vi "Prompt for Step--Init UI.vi"(8 "error in (no error)":errorcluster, 10 "Control Ref Map":map{string, refnum<vi>}(c390), 11 "Timing Action in":refnum<class "Timing Action.lvclass">) -> (0 "error out":errorcluster, 3 "Timing Action out":refnum<class "Timing Action.lvclass">)   [LabVIEW 2020, in "MacroAssert.lvlib" / "Timing Action.lvclass"]
doc: "Initializes the user interface within the \"Prompt for Step\" VI."
uses:
  Timing Action.lvclass
  af30d547-0726-4784-b602-959716fec50c.vi
  bffebe10-a113-4901-af85-4519943715b4.vi
  Support/Get Control Reference by Label (1D STR).vi
  <vilib>/Utility/error.llb/Error Cluster From Error Code.vi
  Action Step/Action Step.lvclass
  MacroAssert.lvlib
  SubVIs/Custom Errors/Custom Errors.lvlib
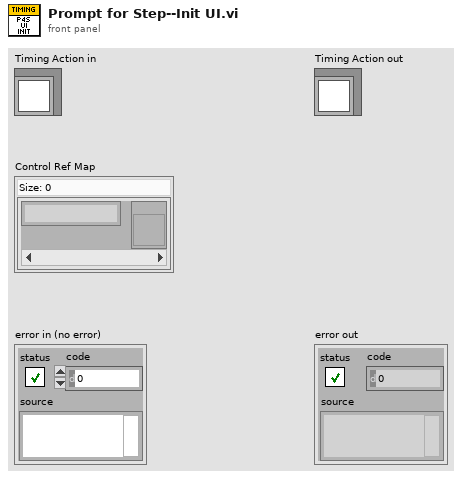
[diagram p1: front panel]
types:
  T1 = typedef "MacroAssert.lvlib/Timing Action.lvclass/Timing Action Type.ctl" = enum16{"Wait", "Wait Until"}
  T2 = typedef "MacroAssert.lvlib/Timing Action.lvclass/Time Unit.ctl" = enum16{"milliseconds", "seconds", "minutes"}
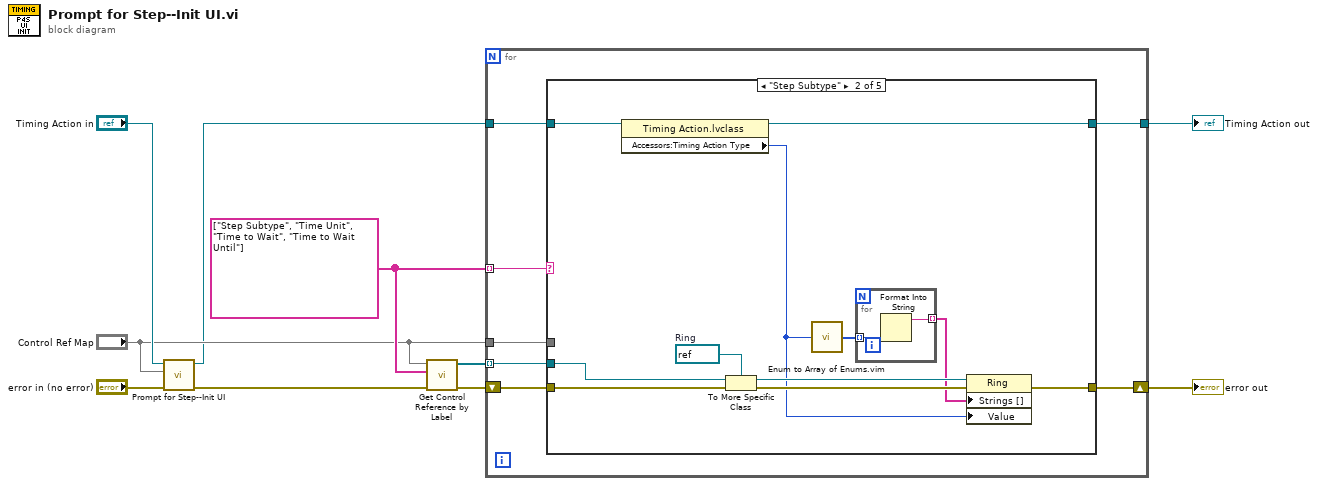
[diagram p0: block diagram]
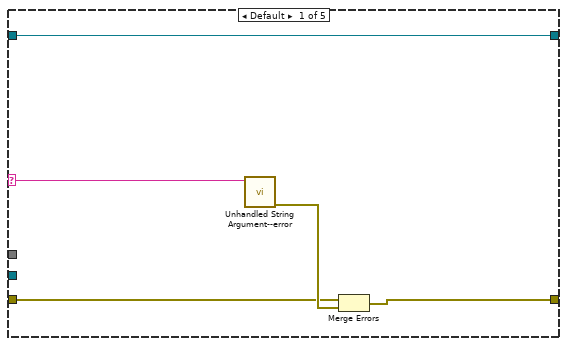
[diagram p2: hidden frame]
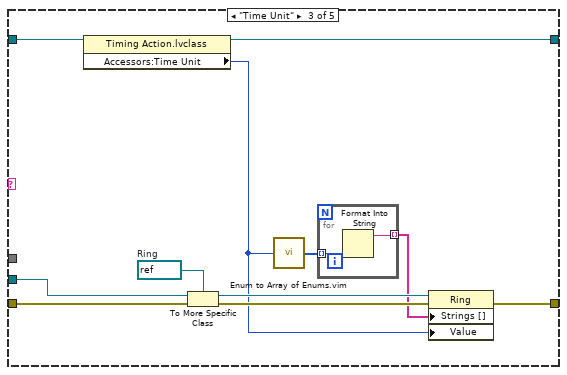
[diagram p3: hidden frame]
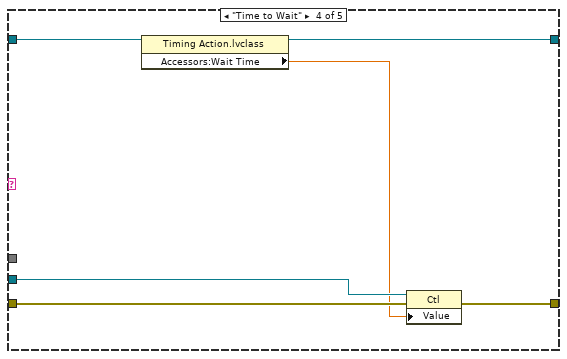
[diagram p4: hidden frame]
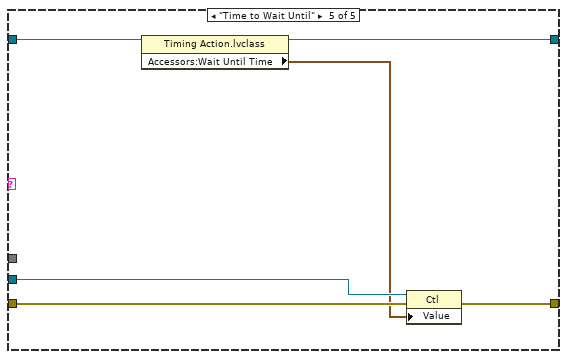
[diagram p5: hidden frame]
diagram:
  w9 = string[] ["Step Subtype", "Time Unit", "Time to Wait", "Time to Wait Until"]
  n1 = call-parent "Prompt for Step--Init UI.vi"("error in (no error)"="error in (no error)", "Control Ref Map"="Control Ref Map", "Step in"="Timing Action in") -> ("error out"=w4:errorcluster, "Step out"=w1:refnum<class "Timing Action.lvclass">)  [unwired: 7 in]
  n2 = call-poly "Get Control Reference by Label.vi"("error in (no error)"=w4, "Control Names"=w9, "Control Ref Map"="Control Ref Map") -> ("error out"=w10:errorcluster, "Control Refs"=w8:refnum<vi>[])  [unwired: 6 in, 1 out]
  n3 = for {
    tunnel: w1 -> [w15]
    tunnel: [w13] -> w5
    tunnel: w9 -> [w16] mode=indexing
    tunnel: w8 -> [w14] mode=indexing
    shift-right: [w12] -> w7
    shift-left: w10 -> [w17]
    tunnel: "Control Ref Map" -> [w11]
    n4 = case shown="\"Step Subtype\"" w16 {
      selector: w16 -> [w18 _ _ _ _]
      tunnel: w17 -> [w20 w26 w39 w51 w57]
      tunnel: w15 -> [w22 w27 w40 w54 w60]
      tunnel: w14 -> [_ w25 w38 w52 w58]
      tunnel: [w22 w23 w36 w53 w59] -> w13
      tunnel: [w19 w24 w37 w49 w55] -> w12
      tunnel: w11 -> [_ _ _ _ _]
      frame Default {
        n5 = call "Unhandled String Argument--error.vi"("Argument"=w18) -> ("error out"=w21:errorcluster)  [unwired: 10 in]
        n6 = Merge Errors(w20, w21) -> (w19:errorcluster)
      }
      frame "Step Subtype" {
        w30 = refnum<vi> refnum  # Ring
        n7 = property class="Timing Action.lvclass"(reference=w27) -> (reference out=w23:refnum<class "Timing Action.lvclass">, "Accessors:Timing Action Type"=w29:T1)  [unwired: 1 in, 1 out]
        n8 = To More Specific Class(target class=w30, reference=w25, error in=w26) -> (specific class reference=w33:refnum<vi>, error out=w31:errorcluster)
        n9 = call "Enum to Array of Enums.vim"("enum"=w29) -> ("array of enums"=w32:T1[])
        n10 = for {
          tunnel: w32 -> [w35] mode=indexing
          tunnel: [w34] -> w28 mode=indexing
          n11 = Format Into String(w35) -> (resulting string=w34:string)  [unwired: 3 in, 1 out]
        }
        n12 = property class="Ring"(reference=w33, error in=w31, "Strings []"=w28, "Value"=w29) -> (error out=w24:errorcluster)  [unwired: 1 out]
      }
      frame "Time Unit" {
        w43 = refnum<vi> refnum  # Ring
        n13 = property class="Timing Action.lvclass"(reference=w40) -> (reference out=w36:refnum<class "Timing Action.lvclass">, "Accessors:Time Unit"=w42:T2)  [unwired: 1 in, 1 out]
        n14 = To More Specific Class(target class=w43, reference=w38, error in=w39) -> (specific class reference=w46:refnum<vi>, error out=w44:errorcluster)
        n15 = call "Enum to Array of Enums.vim"("enum"=w42) -> ("array of enums"=w45:T2[])
        n16 = for {
          tunnel: w45 -> [w48] mode=indexing
          tunnel: [w47] -> w41 mode=indexing
          n17 = Format Into String(w48) -> (resulting string=w47:string)  [unwired: 3 in, 1 out]
        }
        n18 = property class="Ring"(reference=w46, error in=w44, "Strings []"=w41, "Value"=w42) -> (error out=w37:errorcluster)  [unwired: 1 out]
      }
      frame "Time to Wait" {
        n19 = property class="Timing Action.lvclass"(reference=w54) -> (reference out=w53:refnum<class "Timing Action.lvclass">, "Accessors:Wait Time"=w50:dbl)  [unwired: 1 in, 1 out]
        n20 = property class="Ctl"(reference=w52, error in=w51, "Value"=w50) -> (error out=w49:errorcluster)  [unwired: 1 out]
      }
      frame "Time to Wait Until" {
        n21 = property class="Timing Action.lvclass"(reference=w60) -> (reference out=w59:refnum<class "Timing Action.lvclass">, "Accessors:Wait Until Time"=w56:timestamp)  [unwired: 1 in, 1 out]
        n22 = property class="Ctl"(reference=w58, error in=w57, "Value"=w56) -> (error out=w55:errorcluster)  [unwired: 1 out]
      }
    }
  }
  "error out" <- w7
  "Timing Action out" <- w5
